vi "Trav_pos_for_Email.vi"() -> (0 "String":string)   [LabVIEW 2012]
uses:
  Controls/Overhead.ctl
  Globals/Trav_pos_global.vi
  Globals/Meas_global.vi
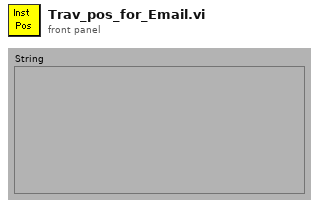
[diagram p1: front panel]
types:
  T1 = typedef "Overhead.ctl" = enum16{"Update total times", "Read Current Overhead", "Re Scale totals to 3 hrs", "Initialise totals to 3hr"}
  T2 = typedef "Tunnel_Coordinates.ctl" = enum16{"Work in Tunnel Coordinates", "Work in Model Coordinates"}
  T3 = typedef "Traverse_cluster.ctl" = cluster{"Start X":dbl, "Start Y":dbl, "Start Z":dbl, "End X":dbl, "End Y":dbl, "End Z":dbl, "No. of pts.":i32, "Spacing":T4, "Filename":path, "Tunnel Speed":dbl, "Averaging time (min)":dbl, "Extra Commands":string, "Specific Arguments":string, "Emission Rate (l/min)":dbl, "Trace Gas Concentration (%)":dbl, "Density Ratio":string, "Comments":string, "Row No":i32, "Row Type Selector":T5, "Completion time":string, "Row Duration (mins)":dbl, "No. of Valid pts.":i32, "Meas Setup File":string}
  T4 = typedef "Spacing.ctl" = enum16{"Linear", "Log", "Gauss", "Specified", "N/A"}
  T5 = typedef "Multi_run_mode.ctl" = enum16{"Move Traverse Only", "Set Tunnel Speed Only", "Set Source Only", "Set Measurement Conditions", "Single Measurement", "Vertical Profile", "Lateral Profile", "Longitudinal Profile", "Explore Volume", "Multi-Axis Profile", "Auto Calibrate", "Meas Fast FID Bkgnd", "Check Beam Power", "Scanning Valve Measurement", "Run VI Named:", "Set ADAM Ch", "Wait (minutes)", "Send Message", "Synchronize With:", "Fall Back to this Row", "Turn Off Row Repeating", "Blank Row", "Traverse 3D Volume"}
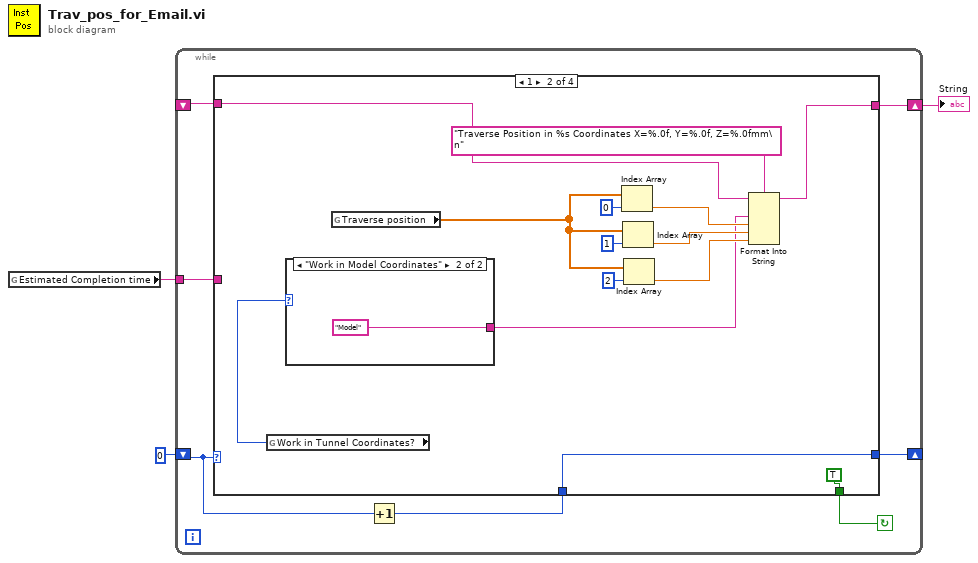
[diagram p0: block diagram]
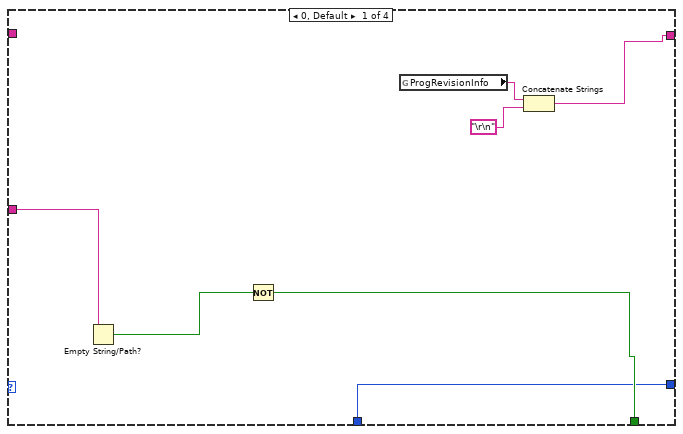
[diagram p2: hidden frame]
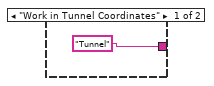
[diagram p3: hidden frame]
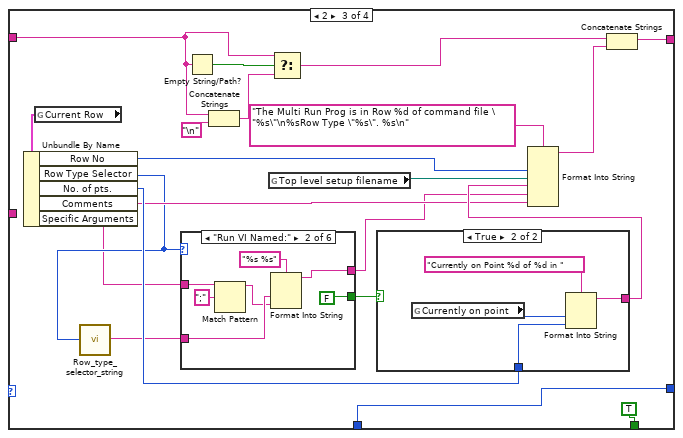
[diagram p4: hidden frame]
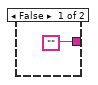
[diagram p5: hidden frame]
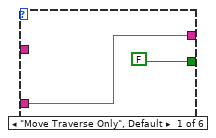
[diagram p6: hidden frame]
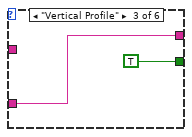
[diagram p7: hidden frame]
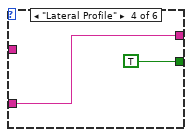
[diagram p8: hidden frame]
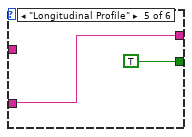
[diagram p9: hidden frame]
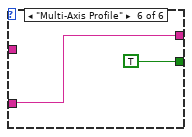
[diagram p10: hidden frame]
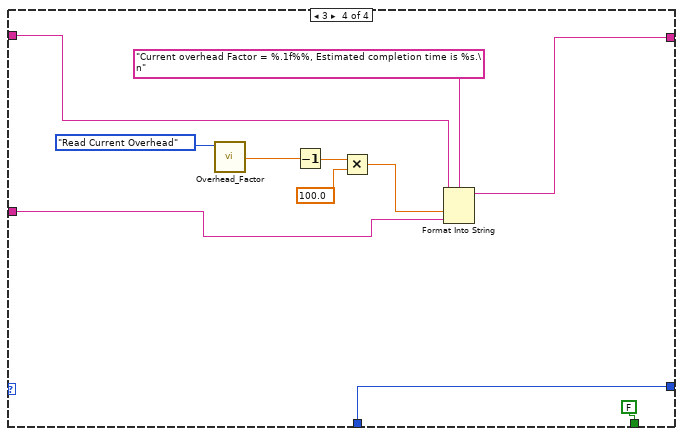
[diagram p11: hidden frame]
diagram:
  n1 = global read "Trav_pos_global.vi" "Estimated Completion time"() -> (w1:string)
  n2 = while {
    shift-left: _ -> [w5]
    shift-right: [w7] -> w2
    shift-left: 0 -> [w10]
    shift-right: [w9] -> _
    tunnel: w1 -> [w4]
    stop <- w6 continue-if-true
    n3 = Increment(x=w10) -> (x+1=w8:i32)
    n4 = case shown="1" w10 {
      tunnel: [w14 w31 w48 w86] -> w9
      tunnel: w8 -> [w14 w31 w48 w86]
      tunnel: [w12 w22 w54 w78] -> w7
      tunnel: [w15 TRUE TRUE FALSE] -> w6
      tunnel: w5 -> [_ w23 w45 w79]
      tunnel: w4 -> [w17 _ _ w77]
      frame 0, Default {
        n5 = Empty String/Path?(string/path=w17) -> (empty?=w16:bool)
        n6 = Not(x=w16) -> (.not. x?=w15:bool)
        n7 = global read "Meas_global.vi" "ProgRevisionInfo"() -> (w13:string)
        n8 = Concatenate Strings(w13, "\r\n") -> (w12:string)
      }
      frame 1 {
        n9 = global read "Trav_pos_global.vi" "Work in Tunnel Coordinates?"() -> (w21:T2)
        n10 = case shown="\"Work in Model Coordinates\"" w21 {
          tunnel: ["Tunnel" "Model"] -> w19
          frame "Work in Tunnel Coordinates" {
          }
          frame "Work in Model Coordinates" {
          }
        }
        n11 = global read "Trav_pos_global.vi" "Traverse position"() -> (w18:dbl[])
        n12 = Index Array(array=w18, index=0) -> (element=w20:dbl)
        n13 = Index Array(array=w18, index=1) -> (element=w25:dbl)
        n14 = Index Array(array=w18, index=2) -> (element=w24:dbl)
        n15 = Format Into String(format string="Traverse Position in %s Coordinates X=%.0f, Y=%.0f, Z=%.0fmm\n" ("Format String"), initial string=w23, w19, w20, w25, w24) -> (resulting string=w22:string)  [unwired: 1 in, 1 out]
      }
      frame 2 {
        n16 = global read "Trav_pos_global.vi" "Current Row"() -> (w39:T3)
        n17 = Unbundle By Name(w39) -> ("Row No"=w53:i32, "Row Type Selector"=w37:T5, "No. of pts."=w51:i32, "Comments"=w38:string, "Specific Arguments"=w34:string)
        n18 = call "Row_type_selector_string.vi"("Mode"=w37) -> ("Output string"=w36:string)
        n19 = case shown="\"Run VI Named:\"" w37 {
          tunnel: [FALSE FALSE TRUE TRUE TRUE TRUE] -> w52
          tunnel: w36 -> [w60 w67 w69 w71 w73 w75]
          tunnel: [w60 w65 w69 w71 w73 w75] -> w35
          tunnel: w34 -> [_ w63 _ _ _ _]
          frame "Move Traverse Only", Default {
          }
          frame "Run VI Named:" {
            n20 = Match Pattern(string=w63, regular expression=";") -> (before substring=w62:string)  [unwired: 4 out]
            n21 = Format Into String(format string="%s %s" ("Format String"), w67, w62) -> (resulting string=w65:string)  [unwired: 2 in, 1 out]
          }
          frame "Vertical Profile" {
          }
          frame "Lateral Profile" {
          }
          frame "Longitudinal Profile" {
          }
          frame "Multi-Axis Profile" {
          }
        }
        n22 = Empty String/Path?(string/path=w45) -> (empty?=w47:bool)
        n23 = Concatenate Strings(w45, "\n") -> (w46:string)
        n24 = global read "Trav_pos_global.vi" "Top level setup filename"() -> (w42:path)
        n25 = Select(t=w45, s=w47, f=w46) -> (s? t:f=w44:string)
        n26 = case shown="True" w52 {
          tunnel: w51 -> [_ w58]
          tunnel: ["" w56] -> w41
          frame False {
          }
          frame True {
            n27 = global read "Trav_pos_global.vi" "Currently on point"() -> (w59:i32)
            n28 = Format Into String(format string="Currently on Point %d of %d in " ("Format String"), w59, w58) -> (resulting string=w56:string)  [unwired: 2 in, 1 out]
          }
        }
        n29 = Format Into String(format string="The Multi Run Prog is in Row %d of command file \"%s\"\n%sRow Type \"%s\". %s\n" ("Format String"), w53, w42, w41, w35, w38) -> (resulting string=w40:string)  [unwired: 2 in, 1 out]
        n30 = Concatenate Strings(w44, w40) -> (w54:string)
      }
      frame 3 {
        n31 = call "Overhead_Factor.vi"("Mode"=Overhead."Read Current Overhead") -> ("Current Overhead Factor"=w84:dbl)  [unwired: 3 in]
        n32 = Decrement(x=w84) -> (x-1=w83:dbl)
        n33 = Multiply(x=w83, y=100.0) -> (x*y=w81:dbl)
        n34 = Format Into String(format string="Current overhead Factor = %.1f%%, Estimated completion time is %s.\n" ("Format String"), initial string=w79, w81, w77) -> (resulting string=w78:string)  [unwired: 1 in, 1 out]
      }
    }
  }
  "String" <- w2
